vi "Apply VNS to Subset of Population.vi"(7 "Max Allowed Time Passed?":bool, 8 "error in (no error)":errorcluster, 9 "Scheduler.lvclass":refnum<class "Scheduler.lvclass">, 10 "GA in":refnum<class "GA.lvclass">, 11 "OSSP_Problem in":refnum<class "OSSP_Problem.lvclass">) -> (0 "error out":errorcluster, 1 "Scheduler.lvclass Out":refnum<class "Scheduler.lvclass">, 2 "GA out":refnum<class "GA.lvclass">, 3 "OSSP_Problem out":refnum<class "OSSP_Problem.lvclass">)   [LabVIEW 2013]
uses:
  Classes/GA.lvclass
  Classes/OSSP_Problem.lvclass
  Classes/Scheduler.lvclass
  Classes/GA.lvclass/GA.ctl
  Classes/Scheduler.lvclass/Scheduler.ctl
  Classes/OSSP_Problem.lvclass/OSSP_Problem.ctl
  Classes/GA_Class/Controls/Solution_GA.ctl
  Insert Neighborhood.vi
  Inversion Neighborhood.vi
  Zobolas Local Search Engine.vi
  Classes/OSSP_Problem_Class/Getters/Read Number of Machines.vi
  Global Schedule Selector.vi
  GA/SubVIS/Remove Duplicates In Array.vi
  Generate Two Indices for Local Search.vi
  Or-Opt(Zobolas) Neighborhood.vi
  Swap Neighborhood.vi
  Classes/Scheduler_Class/NonDelay Scheduler/Non Delay Scheduler Engine.vi
  Classes/OSSP_Problem_Class/Getters/Read Number of Jobs.vi
  Classes/OSSP_Problem_Class/Getters/Read Processing Times.vi
  GA/SubVIS/Calcualte General Tardiness.vi
  Classes/OSSP_Problem_Class/Getters/Read Due Dates.vi
  Classes/Scheduler_Class/Giffler Thompson Active Schedule Engine.vi
  Classes/Scheduler_Class/Prins FIFO Scheduler Methods and Controls/Methods/Calculate Makespan (Prins FIFO Engine).vi
  Classes/Scheduler_Class/Prins FIFO Scheduler Methods and Controls/Methods/Calculate Tardiness (Prins FIFO Engine).vi
  Classes/Scheduler_Class/Modified GT Active Scheduler/GT Active Scheduler wSubset4Tardiness.vi
  Classes/Scheduler_Class/Getters/Read Lambda.vi
  Classes/Scheduler_Class/Getters/Read Operation Selection Rule.vi
  Classes/Scheduler_Class/Getters/Read Scheduler.vi
  Classes/Scheduler_Class/Operation to Machine Job Tuple.vi
  Classes/Scheduler_Class/Prins FIFO Scheduler Methods and Controls/Prins FIFO Scheduler.vi
  Classes/Scheduler_Class/Prins FIFO Scheduler Methods and Controls/Methods/Calculate Final Completion Times of Jobs.vi
  Classes/Scheduler_Class/Prins FIFO Scheduler Methods and Controls/Methods/Reorder Schedule(Prins FIFO) based on Start Times.vi
  Classes/Scheduler_Class/Modified GT Active Scheduler/GT Find Subset of Operations.vi
  Classes/Scheduler_Class/Modified GT Active Scheduler/Select Operation to Schedule Based on Rule.vi
  Classes/Scheduler_Class/Prins FIFO Scheduler Methods and Controls/Methods/UpdateMachineGaps.vi
  Classes/Scheduler_Class/Prins FIFO Scheduler Methods and Controls/Methods/UpdateJobGaps.vi
  Classes/Scheduler_Class/Prins FIFO Scheduler Methods and Controls/Methods/Find Intersecting Gaps.vi
  Classes/Scheduler_Class/GT Algorithm Find M_ok and J_ok.vi
  Classes/Scheduler_Class/Prins FIFO Scheduler Methods and Controls/Methods/Transform to Plain Job and Machine Gaps Array.vi
  Classes/Scheduler_Class/Semiactive Scheduler/Semi Active Scheduler Engine.vi
  Nonredundant Swap Neighborhood.vi
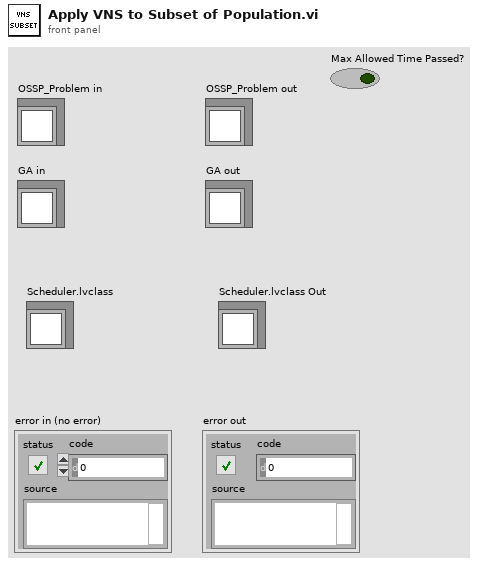
[diagram p1: front panel]
types:
  T1 = typedef "Solution_GA.ctl" = cluster{"Schedule":u16[], "Fitness":u16, "Fitness Valid?":bool}
  T2 = typedef "Objective.ctl" = enum16{"Makespan", "Total Tardiness"}
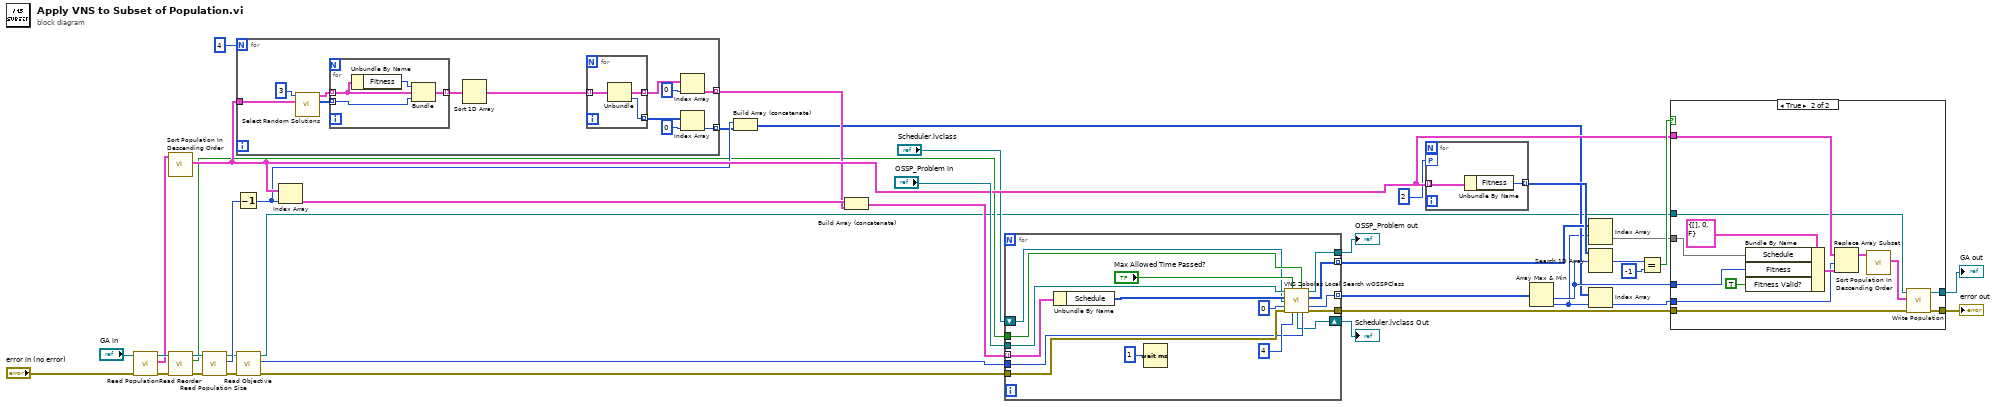
[diagram p0: block diagram]
diagram:
  n1 = call "Read Population.vi"("error in (no error)"="error in (no error)", "GA in"="GA in") -> ("error out"=w30:errorcluster, "Population"=w26:T1[], "GA out"=w29:refnum<class "GA.lvclass">)  [unwired: 7 in]
  n2 = call "Sort Population In Descending Order.vi"("Population"=w26) -> ("Population In Descending Order"=w22:T1[])  [unwired: 9 in, 1 out]
  n3 = call "Read Reorder.vi"("error in (no error)"=w30, "GA in"=w29) -> ("error out"=w25:errorcluster, "Reorder"=w5:bool, "GA out"=w24:refnum<class "GA.lvclass">)  [unwired: 7 in]
  n4 = call "Read Population Size.vi"("error in (no error)"=w25, "GA in"=w24) -> ("error out"=w8:errorcluster, "Population Size"=w23:u8, "GA out"=w7:refnum<class "GA.lvclass">)  [unwired: 7 in]
  n5 = for {
    N: 4 -> [_]
    tunnel: [w46] -> w20 mode=indexing
    tunnel: w22 -> [w44]
    tunnel: [w41] -> w17 mode=indexing
    n6 = call "Select Random Solutions.vi"("Population"=w44, "Tournament Size"=3) -> ("Solution Indices"=w47:i32[], "Selected Solutions"=w51:T1[])  [unwired: 8 in]
    n7 = for {
      tunnel: w51 -> [w58] mode=indexing
      tunnel: [w57] -> w50 mode=indexing
      tunnel: w47 -> [w56] mode=indexing
      n8 = Unbundle By Name(w58) -> ("Fitness"=w59:u16)
      n9 = Bundle("Fitness"=w59, "Solution"=w58, w56) -> (w57:cluster{"Fitness":u16, "Solution":T1, i32})  [unwired: 1 in]
    }
    n10 = Sort 1D Array(array=w50) -> (sorted array=w45:cluster{"Fitness":u16, "Solution":T1, i32}[])
    n11 = for {
      tunnel: w45 -> [w55] mode=indexing
      tunnel: [w54] -> w49 mode=indexing
      tunnel: [w53] -> w42 mode=indexing
      n12 = Unbundle(w55) -> ("Solution"=w54:T1, w53:i32)  [unwired: 1 out]
    }
    n13 = Index Array(array=w49, index=0) -> (element=w46:T1)
    n14 = Index Array(array=w42, index=0) -> (element=w41:i32)
  }
  n15 = Decrement(x=w23) -> (x-1=w18:u8)
  n16 = call "Read Objective .vi"("error in (no error)"=w8, "GA in"=w7) -> ("error out"=w2:errorcluster, "Objective"=w6:T2, "GA out"=w3:refnum<class "GA.lvclass">)  [unwired: 7 in]
  n17 = Index Array(array=w22, index=w18) -> (element=w21:T1)
  n18 = Build Array (concatenate)(w18, w17) -> (w12:i32[])
  n19 = Build Array (concatenate)(w21, w20) -> (w19:T1[])
  n20 = for {
    tunnel: [w72] -> w14 mode=indexing
    tunnel: [w71] -> w16 mode=indexing
    tunnel: w19 -> [w68] mode=indexing
    tunnel: "OSSP_Problem in" -> [w75]
    tunnel: [w74] -> w36
    tunnel: w2 -> [w70]
    tunnel: [w69] -> w35
    tunnel: w6 -> [w63]
    tunnel: w5 -> [w62]
    shift-right: [w60] -> w1
    shift-left: "Scheduler.lvclass" -> [w61]
    n21 = Unbundle By Name(w68) -> ("Schedule"=w67:u16[])
    n22 = Wait (ms)(milliseconds to wait=u32 1) -> ()  [unwired: 1 out]
    n23 = call "VNS Zobolas Local Search wOSSPClass.vi"("OSSP_Problem.lvclass"=w75, "Max Allowed Time Passed?"="Max Allowed Time Passed?", "Reorder?"=w62, "Schedule In"=w67, "Scheduler.lvclass"=w61, "Max Iteration Count"=0, "error in (no error)"=w70, "Number of Neighborhoods"=4, "Objective"=w63) -> ("OSSP_Problem out"=w74:refnum<class "OSSP_Problem.lvclass">, "VNS Result Out"=w72:u16[], "Makespan/Tardiness(FIFO Engine)"=w71:u16, "Scheduler.lvclass Out"=w60:refnum<class "Scheduler.lvclass">, "error out"=w69:errorcluster)  [unwired: 2 in]
  }
  "OSSP_Problem out" <- w36
  "Scheduler.lvclass Out" <- w1
  n24 = for {
    tunnel: w22 -> [w77] mode=indexing
    tunnel: [w76] -> w31 mode=indexing
    workers-P: 2 -> [_]
    n25 = Unbundle By Name(w77) -> ("Fitness"=w76:u16)
  }
  n26 = Array Max & Min(array=w16) -> (min value=w15:u16, min index (indices)=w11:i32)  [unwired: 2 out]
  n27 = Index Array(array=w14, index (row)=w11) -> (element=w13:u16[])  [unwired: 1 in]
  n28 = Search 1D Array(1D array=w31, element=w15) -> (index of element=w34:i32)  [unwired: 1 in]
  n29 = Index Array(array=w12, index=w11) -> (element=w10:i32)
  n30 = Equal?(x=w34, y=-1) -> (x = y?=w28:bool)
  n31 = case shown="True" w28 {
    tunnel: [w79 w92] -> w40
    tunnel: [w78 w91] -> w39
    tunnel: w35 -> [w78 w90]
    tunnel: w22 -> [_ w89]
    tunnel: w3 -> [w79 w88]
    tunnel: w15 -> [_ w84]
    tunnel: w13 -> [_ w83]
    tunnel: w10 -> [_ w82]
    frame False {
    }
    frame True {
      n32 = Bundle By Name(cluster=T1 {"Schedule"=[], "Fitness"=0, "Fitness Valid?"=FALSE} ("Solution"), "Schedule"=w83, "Fitness"=w84, "Fitness Valid?"=TRUE) -> (w85:T1)
      n33 = Replace Array Subset(array=w89, new element=w85, index=w82) -> (w81:T1[])
      n34 = call "Sort Population In Descending Order.vi"("Population"=w81) -> ("Population In Descending Order"=w80:T1[])  [unwired: 9 in, 1 out]
      n35 = call "Write Population.vi"("error in (no error)"=w90, "Population"=w80, "GA in"=w88) -> ("error out"=w91:errorcluster, "GA out"=w92:refnum<class "GA.lvclass">)  [unwired: 7 in]
    }
  }
  "GA out" <- w40
  "error out" <- w39
